vi "problem3-Server.vi"() -> ()   [LabVIEW 2017]
panel:
  out "error out":errorcluster
  in  "Numeric":dbl
  in  "stop":bool
  in  "Numeric 2":dbl
  in  "Numeric 3":dbl
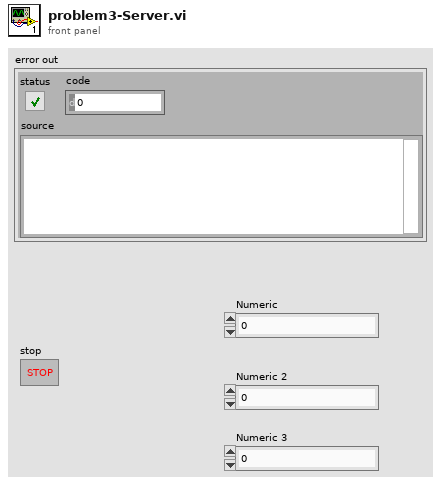
[diagram p1: front panel]
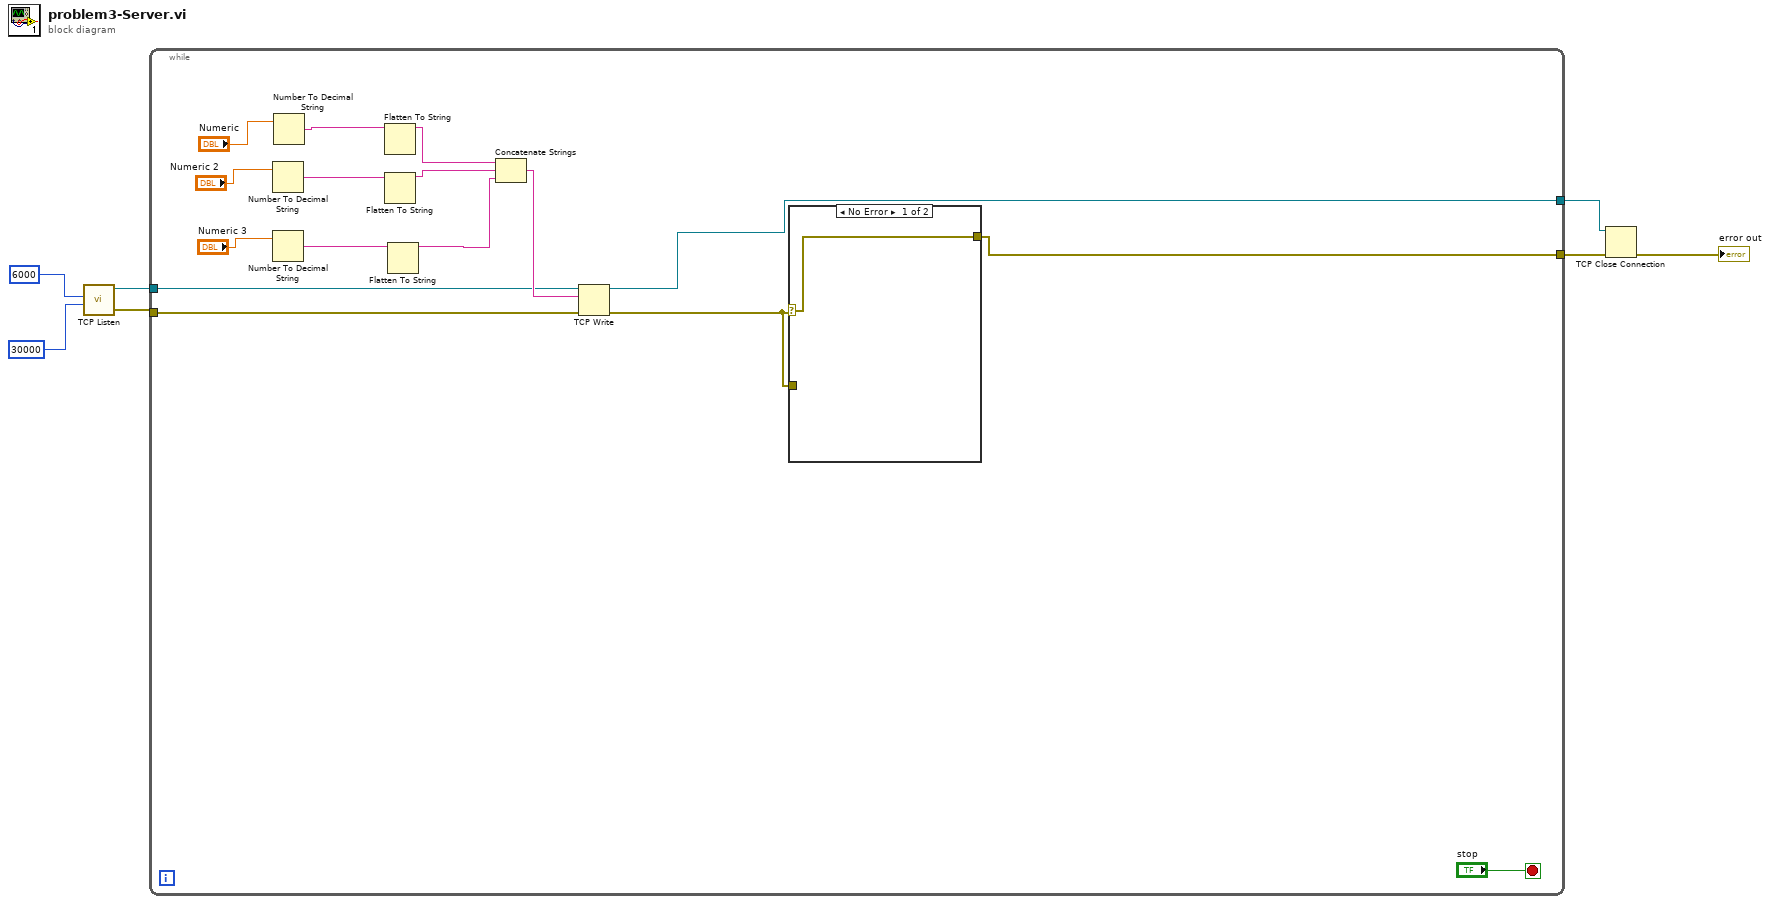
[diagram p0: block diagram]
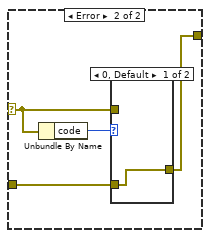
[diagram p2: hidden frame]
diagram:
  n1 = call <vilib>:"TCP Listen.vi"("timeout ms (wait forever: -1)"=30000, "port"=u16 6000) -> ("error out"=w3:errorcluster, "connection ID"=w4:refnum<k5>)  [unwired: 5 in, 3 out]
  n2 = while {
    tunnel: w4 -> [w12]
    tunnel: w3 -> [w11]
    tunnel: [w9] -> w2
    tunnel: [w8] -> w1
    stop <- "stop" stop-if-true
    n3 = Number To Decimal String(number="Numeric 2") -> (decimal integer string=w20:string)  [unwired: 1 in]
    n4 = Number To Decimal String(number="Numeric 3") -> (decimal integer string=w19:string)  [unwired: 1 in]
    n5 = Number To Decimal String(number="Numeric") -> (decimal integer string=w21:string)  [unwired: 1 in]
    n6 = Flatten To String(anything=w21) -> (data string=w18:string)  [unwired: 3 in, 2 out]
    n7 = Flatten To String(anything=w20) -> (data string=w17:string)  [unwired: 3 in, 2 out]
    n8 = Flatten To String(anything=w19) -> (data string=w16:string)  [unwired: 3 in, 2 out]
    n9 = Concatenate Strings(w18, w17, w16) -> (w13:string)
    n10 = TCP Write(connection ID=w12, data in=w13, error in (no error)=w11) -> (connection ID out=w9:refnum<k5>, error out=w10:errorcluster)  [unwired: 1 in, 1 out]
    n11 = case shown="No Error" w10 {
      selector: w10 -> [w24 w27]
      tunnel: [w24 w25] -> w8
      tunnel: w10 -> [_ w26]
      frame No Error {
      }
      frame Error {
        n12 = Unbundle By Name(w27) -> ("code"=w28:i32)
        n13 = case shown="0, Default" w28 {
          tunnel: w27 -> [_ _]
          tunnel: w26 -> [w29 w30]
          tunnel: [w29 w30] -> w25
          frame 0, Default {
          }
          frame 56 {
          }
        }
      }
    }
  }
  n14 = TCP Close Connection(connection ID=w2, error in (no error)=w1) -> (error out=→"error out":errorcluster)  [unwired: 1 in, 1 out]
